vi "Clear FFT Evaluated Waveform Count.vi"(8 "error in (no error)":errorcluster, 11 "VISA resource name":refnum<visa-resource-name>) -> (0 "error out":errorcluster, 3 "VISA resource name out":refnum<visa-resource-name>)   [LabVIEW 2015, in "Agilent 2000 3000 X-Series.lvlib"]
doc: "Clears the number of evaluated waveforms, when the FFT display mode is AVERage, MAXHold, or MINHold\n\nNotes:\nOnly supported by the 3000 T Series."
uses:
  Agilent 2000 3000 X-Series.lvlib
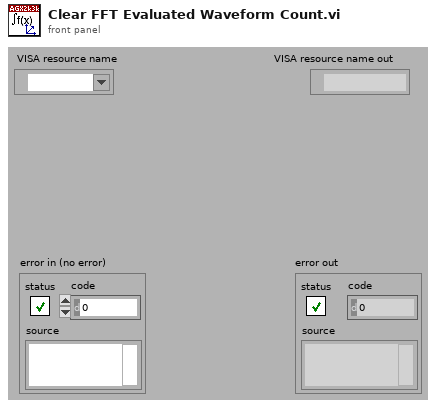
[diagram p1: front panel]
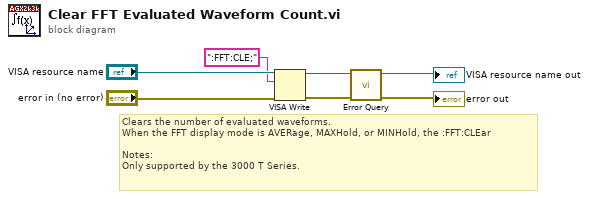
[diagram p0: block diagram]
diagram:
  # "Clears the number of evaluated waveforms.\nWhen the FFT display mode is AVERage, MAXHold, or MINHold, the :FFT:CLEar\n\nNotes:\nOnly supported by the 3000 T Series."
  n1 = VISA Write(VISA resource name="VISA resource name", write buffer=":FFT:CLE;", error in (no error)="error in (no error)") -> (VISA resource name out=w7:refnum<visa-resource-name>, error out=w6:errorcluster)  [unwired: 1 out]
  n2 = call "Error Query.vi"("error in (no error)"=w6, "VISA resource name"=w7) -> ("error out"=→"error out":errorcluster, "VISA resource name out"=→"VISA resource name out":refnum<visa-resource-name>)  [unwired: 8 out]
